vi "WriteData.vi"(8 "Error In":errorcluster, 10 "Data":string, 11 "reference in":refnum<class "FileDataSource.lvclass">) -> (0 "Error Out":errorcluster, 3 "reference out":refnum<class "FileDataSource.lvclass">)   [LabVIEW 2020, in "FileDataSource.lvclass"]
uses:
  FileDataSource.lvclass
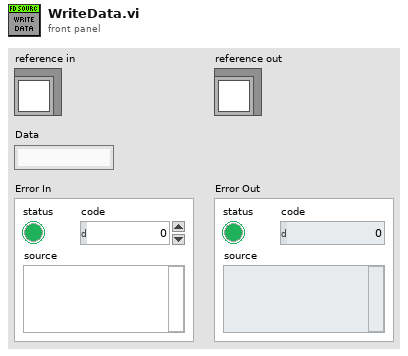
[diagram p1: front panel]
types:
  T1 = typedef "FileDataSource.lvclass/ObjectAttributes.ctl" = cluster{"Name":string}
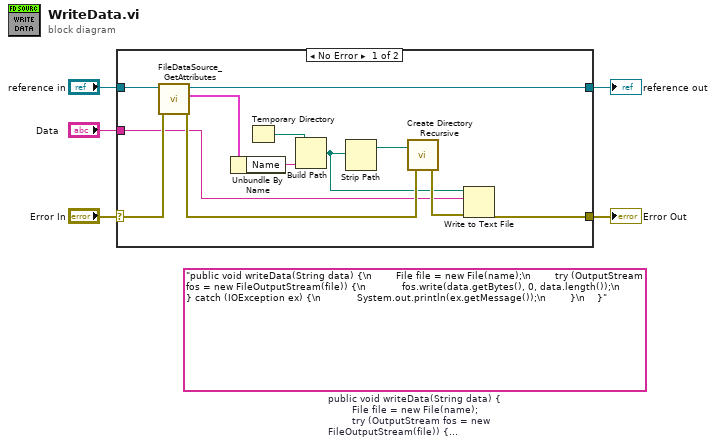
[diagram p0: block diagram]
diagram:
  (unwired) "public void writeData(String data) {\n        File file = new File(name);\n        try (OutputStream fos = new FileOutputStream(file)) {\n            fos.write(data.getBytes(), 0, data.length());\n        } catch (IOException ex) {\n            System.out.println(ex.getMessage());\n        }\n    }"  # public void writeData(String data) {         File file = new File(name);         try (OutputStream fos = new FileOutputStream(file)) {             fos.write(data.getBytes(), 0, data.length());         } catch (IOException ex) {             System.out.println(ex.getMessage());         }     }
  n1 = case shown="No Error" "Error In" {
    selector: "Error In" -> [w16 w19]
    tunnel: [w6 w19] -> w4
    tunnel: [w15 w18] -> w2
    tunnel: "reference in" -> [w17 w18]
    tunnel: "Data" -> [w7 _]
    frame No Error {
      n2 = call "FileDataSource_GetAttributes.vi"("error in (no error)"=w16, "reference in"=w17) -> ("error out"=w10:errorcluster, "Data"=w12:T1, "reference out"=w15:refnum<class "FileDataSource.lvclass">)  [unwired: 6 in, 1 out]
      n3 = Unbundle By Name(w12) -> ("Name"=w14:string)
      n4 = Temporary Directory() -> (w13:path)
      n5 = Build Path(base path=w13, name or relative path=w14) -> (appended path=w8:path)
      n6 = Strip Path(path=w8) -> (stripped path=w11:path)  [unwired: 1 out]
      n7 = call <vilib>:"Create Directory Recursive.vi"("error in (no error)"=w10, "directory"=w11) -> ("error out"=w9:errorcluster)  [unwired: 3 in, 2 out]
      n8 = Write to Text File(file (use dialog)=w8, text=w7, error in=w9) -> (error out=w6:errorcluster)  [unwired: 1 in, 2 out]
    }
    frame Error {
    }
  }
  "Error Out" <- w4
  "reference out" <- w2
